vi "Average_of_Three.vi"(9 "Test 3":dbl, 10 "Test 2":dbl, 11 "Test 1":dbl) -> (3 "Average":dbl)   [LabVIEW 2025]
doc: "Returns the average value of its inputs."
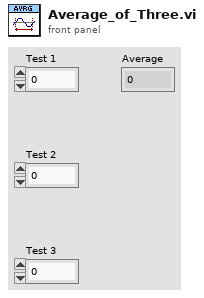
[diagram p1: front panel]
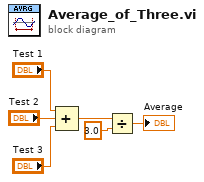
[diagram p0: block diagram]
diagram:
  n1 = Compound Arithmetic op=ADD("Test 1", "Test 2", "Test 3") -> (w4:dbl)
  n2 = Divide(x=w4, y=3.0) -> (x/y=→"Average":dbl)
